vi "Global Limite de test.vi"() -> ()   [LabVIEW 2020]
panel:
  out "Current":dbl
  out "DcirMax":dbl
  out "DeltaTcell 3":dbl
  out "Tcellmax 3":dbl
  out "Tcellmin 3":dbl
  out "DeltaVcell 3":dbl
  out "Vcellmax 3":dbl
  out "Vcellmin 3":dbl
  out "DeltaTcell 2":dbl
  out "Tcellmax 2":dbl
  out "Tcellmin 2":dbl
  out "DeltaVcell 2":dbl
  out "Vcellmax 2":dbl
  out "Vcellmin 2":dbl
  out "Topologie":dbl
  out "Type":dbl
  out "id":dbl
  out "ISO-":dbl
  out "ISO+":dbl
  out "DeltaTcell":dbl
  out "Tcellmax":dbl
  out "Tcellmin":dbl
  out "DeltaVcell":dbl
  out "Vcellmax":dbl
  out "Vcellmin":dbl
  out "ACIRmax":dbl
  out "ACIRmin":dbl
  out "OCVmax":dbl
  out "OCVmin":dbl
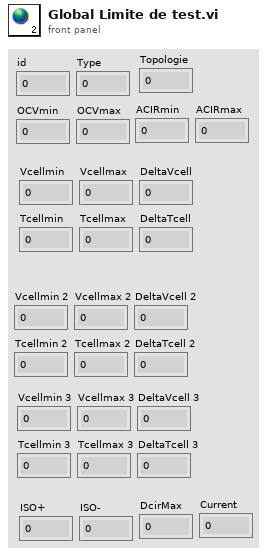
[diagram p1: front panel]
diagram:
